vi "1_Dataset_Generation.vi"() -> ()   [LabVIEW 2020]
doc: "This is a utility VI for synthetic dataset generation based on sample objects and background image for object detection task.\nRequirements: \n1. Deep Learning Toolkit for LabVIEW.\n2. NI Vision Development Module."
uses:
  Controls/Analog_Meter.ctl
  <vilib>/Analysis/1siggen.llb/Ramp Pattern by Samples.vi
  <vilib>/Utility/file.llb/Write Delimited Spreadsheet (string).vi
  <vilib>/vision/NI_Vision_Development_Module.lvlib
  <vilib>/Analysis/NI_AALBase.lvlib
panel:
  out "Status":string="Generating Train Dataset"
  out "Progress":i32=392
  in  "No of Images [Train, Test]":i32[](array[numeric])=[1000, 200]
  in  "Datasets Destination Folder":path=path "D:/DeepLTK_Examples/Analog_Meter"
  in  "Image Resolution":i32=256
  out "Gauge":T1 scale=0.0..140.0
  # "Overview:  This is a utility VI for synthetic dataset generation based on a sample LabVIEW Control.\nThis VI will generate both Train and Test Dataset with specified number of images.\nRequirements: \n1. NI Vision Development Module.\nInstructions:\n1. Provide destination path for datasets to be generated at \"Destination Path for Images(Folder)\".\n2. Run the VI.\n3. Observe the content at destination folder."
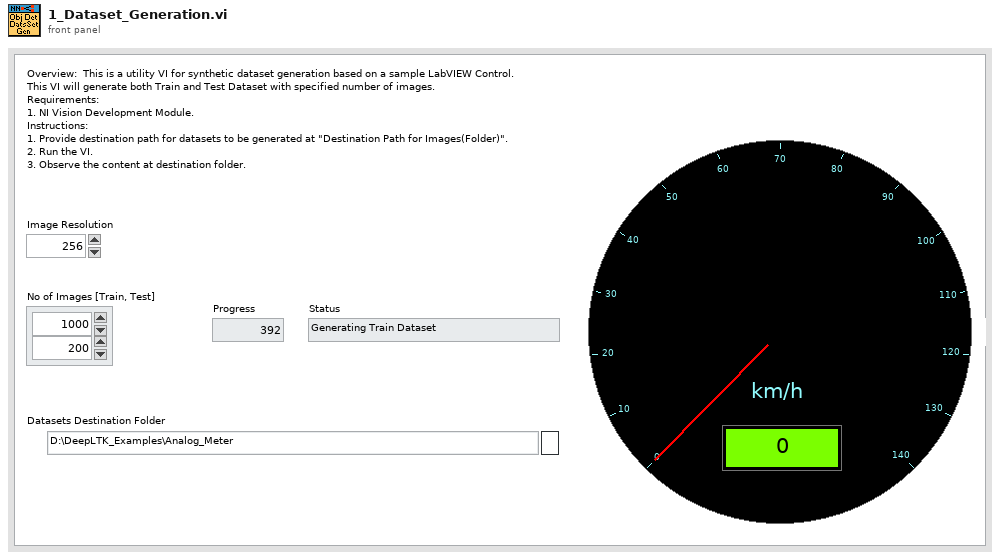
[diagram p1: front panel]
types:
  T1 = typedef "Analog_Meter.ctl" = dbl
  T2 = typedef "Image Type" = u32
  T3 = typedef "IMAQ Image.ctl" = refnum<image>
  T4 = typedef "imagedata.ctl" = cluster{"image type":i32, "image depth":i32, "image":u8[], "mask":u8[], "colors":u32[], "Rectangle":cluster{"left":i16, "top":i16, "right":i16, "bottom":i16}}
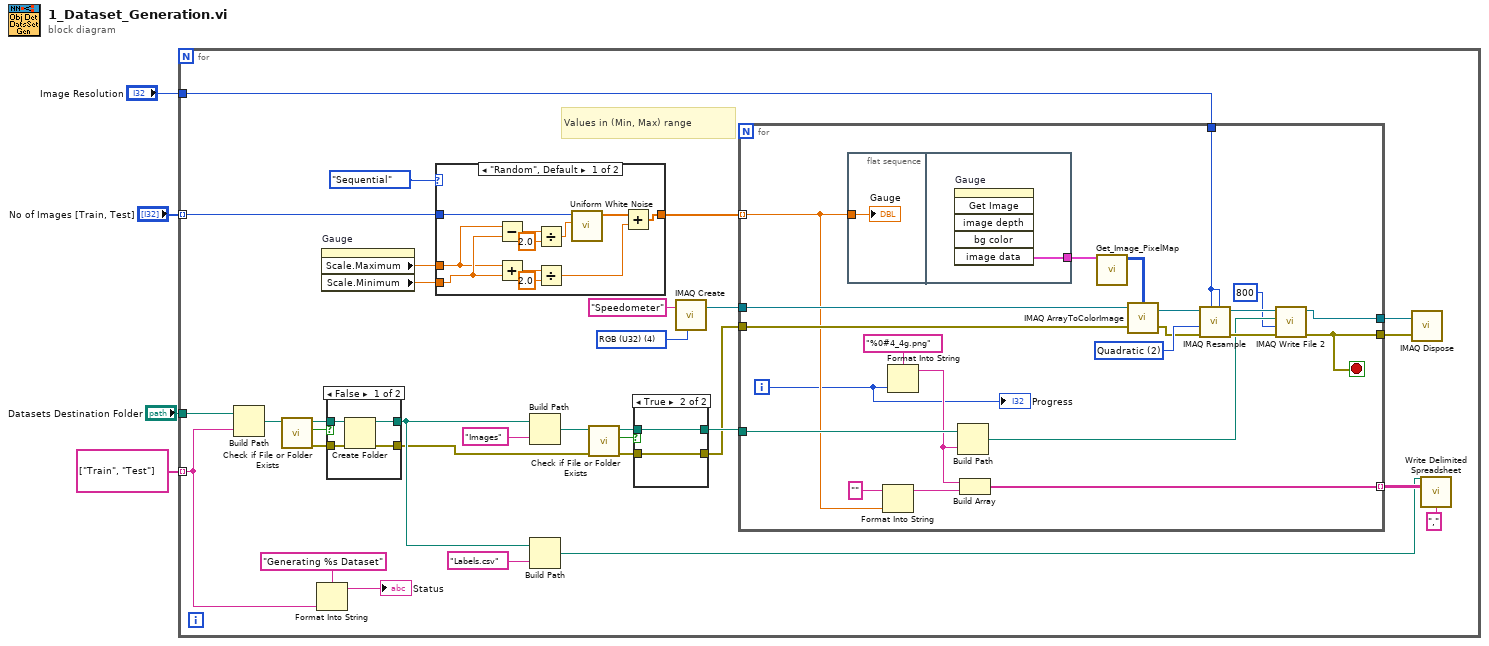
[diagram p0: block diagram]
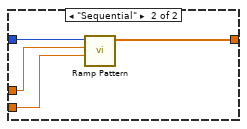
[diagram p2: hidden frame]
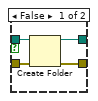
[diagram p3: hidden frame]
diagram:
  n1 = for {
    tunnel: "Datasets Destination Folder" -> [w15]
    tunnel: string[] ["Train", "Test"] ("initial string") -> [w8] mode=indexing
    tunnel: "No of Images [Train, Test]" -> [w12] mode=indexing
    tunnel: "Image Resolution" -> [w11]
    w35 = T2 4 items=["Grayscale (U8)", "Grayscale (I16)", "Grayscale (SGL)", "Complex (CSG)", "RGB (U32)", "HSL (U32)", "RGB (U64)", "Grayscale (U16)"] ("Image Type")
    # "Values in (Min, Max) range"
    n2 = Build Path(base path=w15, name or relative path=w8) -> (appended path=w16:path)
    n3 = call <vilib>:"Check if File or Folder Exists.vi"("path"=w16) -> ("error out"=w18:errorcluster, "file or folder exists?"=w19:bool, "dup path"=w17:path)  [unwired: 8 in]
    n4 = Format Into String(format string="Generating %s Dataset" ("Status"), w8) -> (resulting string=→"Status":string)  [unwired: 2 in, 1 out]
    n5 = property on="Gauge" class="Knob (strict)"() -> ("Scale.Maximum"=w6:dbl, "Scale.Minimum"=w7:dbl)  [unwired: 2 in, 2 out]
    n6 = case shown="False" w19 {
      tunnel: [w85 w87] -> w14
      tunnel: [w84 w86] -> w13
      tunnel: w17 -> [w83 w87]
      tunnel: w18 -> [w82 w86]
      frame False {
        n7 = Create Folder(path (use dialog)=w83, error in=w82) -> (created path=w85:path, error out=w84:errorcluster)  [unwired: 1 in, 1 out]
      }
      frame True {
      }
    }
    n8 = case shown="\"Random\", Default" enum16{"Random", "Sequential"}."Sequential" {
      tunnel: [w45 w48] -> w20
      tunnel: w12 -> [w44 w49]
      tunnel: w7 -> [w39 w51]
      tunnel: w6 -> [w38 w50]
      frame "Random", Default {
        n9 = Subtract(x=w38, y=w39) -> (x-y=w47:dbl)
        n10 = Add(x=w38, y=w39) -> (x+y=w40:dbl)
        n11 = Divide(x=w47, y=2.0) -> (x/y=w42:dbl)
        n12 = Divide(x=w40, y=2.0) -> (x/y=w37:dbl)
        n13 = call <vilib>:"Uniform White Noise.vi"("amplitude"=w42, "samples"=w44) -> ("uniform white noise"=w46:dbl[])  [unwired: 8 in, 1 out]
        n14 = Add(x=w46, y=w37) -> (x+y=w45:dbl[])
      }
      frame "Sequential" {
        n15 = call-poly <vilib>:"Ramp Pattern.vi"("start"=w51, "end"=w50, "samples"=w49) -> ("Ramp Pattern"=w48:dbl[])  [unwired: 7 in, 1 out]
      }
    }
    n16 = Build Path(base path=w14, name or relative path="Images" ("initial string")) -> (appended path=w29:path)
    n17 = Build Path(base path=w14, name or relative path="Labels.csv" ("initial string")) -> (appended path=w25:path)
    n18 = call <vilib>:"Check if File or Folder Exists.vi"("error in (no error)"=w13, "path"=w29) -> ("error out"=w22:errorcluster, "file or folder exists?"=w21:bool, "dup path"=w23:path)  [unwired: 7 in]
    n19 = case shown="True" w21 {
      tunnel: [w79 w81] -> w28
      tunnel: [w78 w80] -> w24
      tunnel: w23 -> [w77 w81]
      tunnel: w22 -> [w76 w80]
      frame False {
        n20 = Create Folder(path (use dialog)=w77, error in=w76) -> (created path=w79:path, error out=w78:errorcluster)  [unwired: 1 in, 1 out]
      }
      frame True {
      }
    }
    n21 = call "IMAQ Create"("Image Name"="Speedometer", "Image Type"=w35) -> ("New Image"=w34:T3)  [unwired: 3 in, 1 out]
    n22 = for {
      tunnel: [w67] -> w36
      tunnel: w28 -> [w66]
      tunnel: w11 -> [w68]
      tunnel: w34 -> [w61]
      tunnel: [w63] -> w33 mode=indexing
      tunnel: [w58] -> w30
      tunnel: w24 -> [w55]
      tunnel: w20 -> [w53] mode=indexing
      i -> [w52]
      stop <- w67 stop-if-true
      w73 = u32 2 items=["Zero Order", "Bi-Linear", "Quadratic", "Cubic Spline"] ("Interpolation Type")
      n23 = flat-sequence {
        tunnel: w53 -> [w74]
        tunnel: [w75] -> w56
        frame #0 {
          "Gauge" <- w74
        }
        frame #1 {
          n24 = invoke on="Gauge" class="Knob (strict)" method="Get Image"() -> ("image data"=w75:T4)  [unwired: 6 in, 5 out]
        }
      }
      n25 = Format Into String(initial string="", w53) -> (resulting string=w62:string)  [unwired: 2 in, 1 out]
      n26 = Format Into String(format string="%0#4_4g.png" ("initial string"), w52) -> (resulting string=w65:string)  [unwired: 2 in, 1 out]
      n27 = Build Path(base path=w66, name or relative path=w65) -> (appended path=w69:path)
      n28 = Build Array(w65, w62) -> (w63:string[])
      n29 = call "Get_Image_PixelMap.vi"("Image Data"=w56) -> ("Image PixelMap"=w59:u32[][])  [unwired: 10 in]
      n30 = call "IMAQ ArrayToColorImage"("Image Pixels (U32)"=w59, "Image"=w61, "error in (no error)"=w55) -> ("Image Out"=w60:T3, "error out"=w54:errorcluster)  [unwired: 2 in]
      n31 = call "IMAQ Resample"("X Resolution"=w68, "Y Resolution"=w68, "error in (no error)"=w54, "Interpolation Type"=w73, "Image Src"=w60) -> ("error out"=w71:errorcluster, "Image Dst Out"=w72:T3)  [unwired: 5 in]
      n32 = call-poly "IMAQ Write File 2"("error in (no error)"=w71, "Image Quality"=u32 800, "File Path"=w69, "Image"=w72) -> ("error out"=w67:errorcluster, "Image Out (duplicate)"=w58:T3)  [unwired: 6 in]
      "Progress" <- w52
    }
    n33 = call "IMAQ Dispose"("Image"=w30, "error in (no error)"=w36) -> ()  [unwired: 4 in, 1 out]
    n34 = call-poly <vilib>:"Write Delimited Spreadsheet.vi"("file path (dialog if empty)"=w25, "2D data"=w33, "delimiter (\\t)"="," ("delimiter (\\t)")) -> ()  [unwired: 11 in, 2 out]
  }
